vi "FT10_M4X Single Capture with Autoscale.vi"(9 "memsize":i32=16384, 10 "Sample Rate (Hz)":i32=130000000, 11 "Card Handle in":u32) -> (2 "Data":waveform(sgl)[](graph), 3 "Card Handle out":u32)   [LabVIEW 2024]
doc: "Copy of \"M4X_Single Capture with Autoscale.vi\" from HWT_Lillis_7854.lvproj"
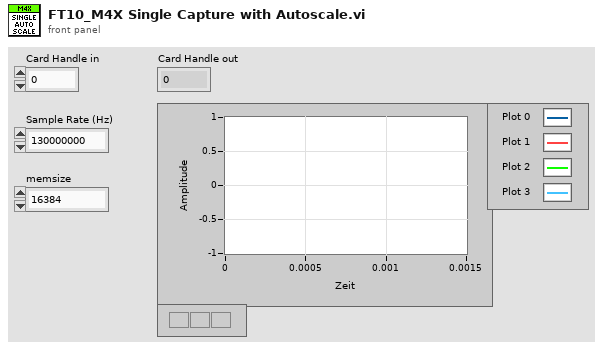
[diagram p1: front panel]
types:
  T1 = enum16{"+/- 200 mV", "+/- 500 mV", "+/- 1 V", "+/- 2 V", "+/- 5 V", "+/- 10 V"}
  T2 = enum16{"+/- 200 mV", "+/- 500 mV", "+/- 1 V", "+/- 2 V", "+/- 5 V", "+/- 10 V"}[]
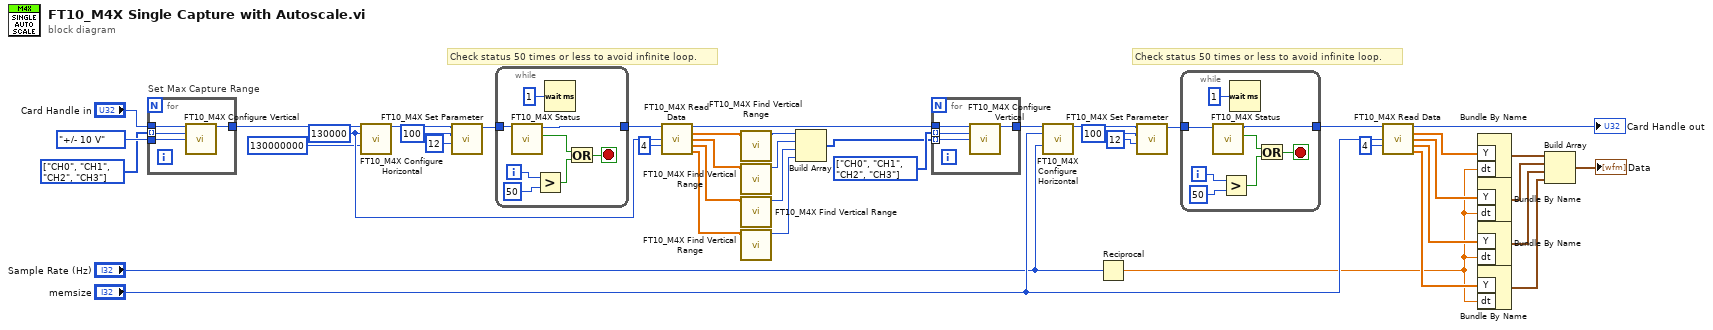
[diagram p0: block diagram]
diagram:
  w9 = enum16{"CH0", "CH1", "CH2", "CH3"}[] [enum."CH0", enum."CH1", enum."CH2", enum."CH3"] items=["CH0", "CH1", "CH2", "CH3"]
  w8 = enum16{"CH0", "CH1", "CH2", "CH3"}[] [enum."CH0", enum."CH1", enum."CH2", enum."CH3"] items=["CH0", "CH1", "CH2", "CH3"]
  w19 = 130000 ("memsize")
  # "Check status 50 times or less to avoid infinite loop."
  # "Check status 50 times or less to avoid infinite loop."
  n1 = for "Set Max Capture Range" {
    tunnel: T1."+/- 10 V" ("Range") -> [w45]
    tunnel: "Card Handle in" -> [w47]
    tunnel: [w44] -> w12
    tunnel: w9 -> [w46] mode=indexing
    n2 = call "FT10_M4X Configure Vertical.vi"("Card Handle in"=w47, "Channel"=w46, "Range"=w45) -> ("Card Handle out"=w44:u32)  [unwired: 11 in, 1 out]
  }
  n3 = call "FT10_M4X Configure Horizontal.vi"("Card Handle in"=w12, "memsize"=w19, "sample rate (Hz)"=130000000) -> ("Card Handle out"=w14:u32)  [unwired: 11 in, 1 out]
  n4 = call "FT10_M4X Set Parameter.vi"("Value"=12, "Register"=100, "Card Handle in"=w14) -> ("Card Handle out"=w17:u32)  [unwired: 7 in, 1 out]
  n5 = while {
    tunnel: w17 -> [w54]
    tunnel: [w53] -> w18
    i -> [w52]
    stop <- w50 stop-if-true
    n6 = call "FT10_M4X Status.vi"("Card Handle in"=w54) -> ("Ready?"=w48:bool, "Card Handle out"=w53:u32)  [unwired: 9 in]
    n7 = Greater?(x=w52, y=50) -> (0:w49:bool)
    n8 = Wait (ms)(milliseconds to wait=u32 1) -> ()  [unwired: 1 out]
    n9 = Or(x=w48, y=w49) -> (x .or. y?=w50:bool)
  }
  n10 = call "FT10_M4X Read Data.vi"("Card Handle in"=w18, "Length (Samples per Channel)"=w19, "Channel Count"=u32 4) -> ("Card Handle out"=w21:u32, "Ch 0"=w22:sgl[], "Ch 1"=w23:sgl[], "Ch 2"=w24:sgl[], "Ch 3"=w25:sgl[])  [unwired: 8 in]
  n11 = call "FT10_M4X Find Vertical Range.vi"("Sample"=w22) -> ("Range"=w26:T1)  [unwired: 10 in]
  n12 = call "FT10_M4X Find Vertical Range.vi"("Sample"=w23) -> ("Range"=w27:T1)  [unwired: 10 in]
  n13 = call "FT10_M4X Find Vertical Range.vi"("Sample"=w24) -> ("Range"=w28:T1)  [unwired: 10 in]
  n14 = call "FT10_M4X Find Vertical Range.vi"("Sample"=w25) -> ("Range"=w29:T1)  [unwired: 10 in]
  n15 = Build Array(w26, w27, w28, w29) -> (w7:T2)
  n16 = for {
    tunnel: w7 -> [w57] mode=indexing
    tunnel: w21 -> [w59]
    tunnel: [w56] -> w30
    tunnel: w8 -> [w58] mode=indexing
    n17 = call "FT10_M4X Configure Vertical.vi"("Card Handle in"=w59, "Channel"=w58, "Range"=w57) -> ("Card Handle out"=w56:u32)  [unwired: 11 in, 1 out]
  }
  n18 = call "FT10_M4X Configure Horizontal.vi"("Card Handle in"=w30, "memsize"="memsize", "sample rate (Hz)"="Sample Rate (Hz)") -> ("Card Handle out"=w32:u32)  [unwired: 11 in, 1 out]
  n19 = Reciprocal(x="Sample Rate (Hz)") -> (1/x=w4:dbl)
  n20 = call "FT10_M4X Set Parameter.vi"("Value"=12, "Register"=100, "Card Handle in"=w32) -> ("Card Handle out"=w35:u32)  [unwired: 7 in, 1 out]
  n21 = while {
    tunnel: w35 -> [w66]
    tunnel: [w65] -> w36
    i -> [w62]
    stop <- w61 stop-if-true
    n22 = call "FT10_M4X Status.vi"("Card Handle in"=w66) -> ("Ready?"=w64:bool, "Card Handle out"=w65:u32)  [unwired: 9 in]
    n23 = Greater?(x=w62, y=50) -> (0:w60:bool)
    n24 = Wait (ms)(milliseconds to wait=u32 1) -> ()  [unwired: 1 out]
    n25 = Or(x=w64, y=w60) -> (x .or. y?=w61:bool)
  }
  n26 = call "FT10_M4X Read Data.vi"("Card Handle in"=w36, "Length (Samples per Channel)"="memsize", "Channel Count"=u32 4) -> ("Card Handle out"=→"Card Handle out":u32, "Ch 0"=w38:sgl[], "Ch 1"=w39:sgl[], "Ch 2"=w40:sgl[], "Ch 3"=w41:sgl[])  [unwired: 8 in]
  n27 = Bundle By Name("Y"=w38, "dt"=w4) -> (w1:waveform(sgl))  [unwired: 1 in]
  n28 = Bundle By Name("Y"=w39, "dt"=w4) -> (w2:waveform(sgl))  [unwired: 1 in]
  n29 = Bundle By Name("Y"=w40, "dt"=w4) -> (w5:waveform(sgl))  [unwired: 1 in]
  n30 = Bundle By Name("Y"=w41, "dt"=w4) -> (w6:waveform(sgl))  [unwired: 1 in]
  n31 = Build Array(w1, w2, w5, w6) -> (→"Data":waveform(sgl)[])
